vi "CreerReference.vi"() -> ()   [LabVIEW 2012]
panel:
  in  "Numéro":i32
  in  "stop":bool
  in  "Adresse du PilMOT":string="ni.var.psp://localhost/OPC/OPC1/esbimETH_1"
  in  "Move to ref":bool
  in  "Set":bool
  out "error out":errorcluster caption="sortie d'erreur"
  in  "error in (no error)":errorcluster caption="entrée d'erreur (pas d'erreur)"
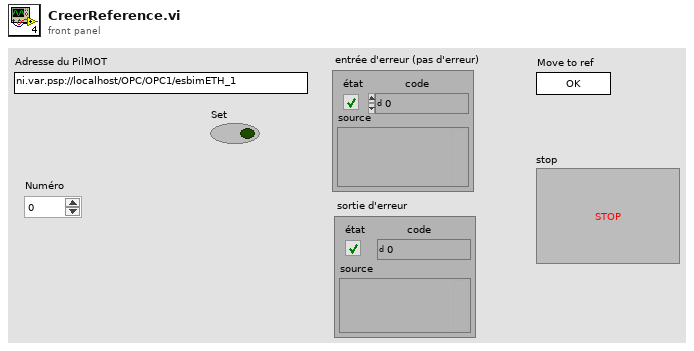
[diagram p1: front panel]
types:
  T1 = typedef "AdressesVariablesPartagees.ctl" = cluster{"OrdreBloc":string, "Ordre UC":string, "CoteAAtteindre":string, "Vitesse":string, "Position codeur en pas":string, "Position Théorique":string, "Message":string, "Ecrire":string, "Zone à écrire":string, "Numéro paramètre":string, "Ordre":string, "Valeur":string, "Valeur Lecture":string, "Numéro paramètre Lecture":string, "Acquittement Lecture Ecriture":string, "Zone à Ecrire Pour Axe ":u16, "Acquittement Ordre UC":string}
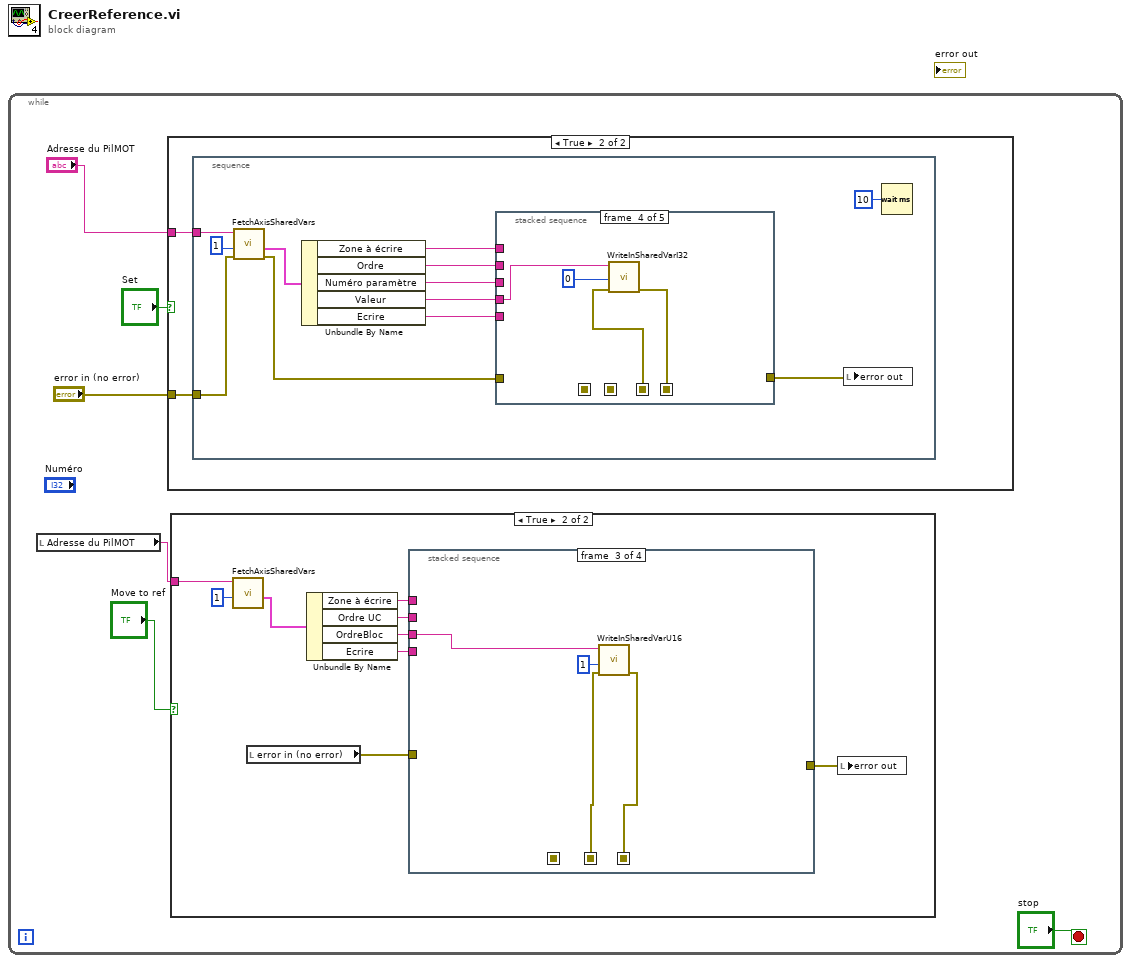
[diagram p0: block diagram]
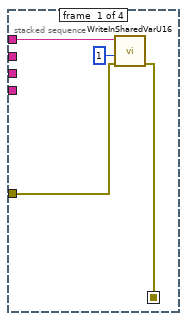
[diagram p3: hidden frame]
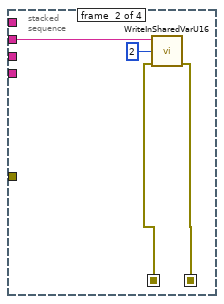
[diagram p4: hidden frame]
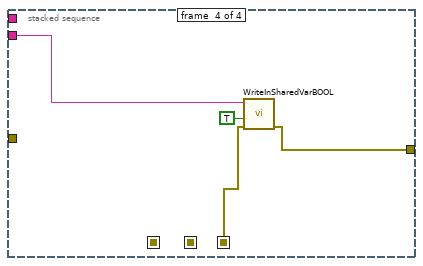
[diagram p5: hidden frame]
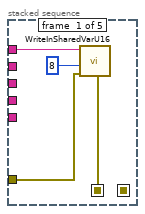
[diagram p7: hidden frame]
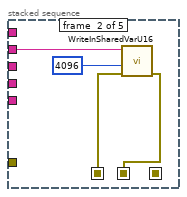
[diagram p8: hidden frame]
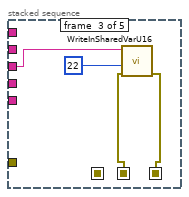
[diagram p9: hidden frame]
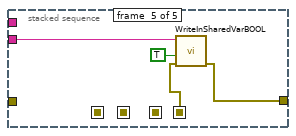
[diagram p10: hidden frame]
diagram:
  n1 = while {
    stop <- "stop" stop-if-true
    n2 = local read "Adresse du PilMOT"() -> (w2:string)
    n3 = case shown="True" "Set" {
      tunnel: "error in (no error)" -> [_ w33]
      tunnel: "Adresse du PilMOT" -> [_ w32]
      frame False {
      }
      frame True {
        n4 = stacked-sequence {
          tunnel: w33 -> [w45]
          tunnel: w32 -> [w44]
          frame #0 {
            n5 = call "FetchAxisSharedVars.vi"("error in (no error)"=w45, "Numéro d'Axe"=u32 1, "PilMOT Address"=w44) -> ("error out"=w36:errorcluster, "Sortie Variables d'Axes"=w37:T1)  [unwired: 7 in]
            n6 = Unbundle By Name(w37) -> ("Zone à écrire"=w43:string, "Ordre"=w42:string, "Numéro paramètre"=w41:string, "Valeur"=w40:string, "Ecrire"=w39:string)
            n7 = stacked-sequence {
              seq-local: [w47 _ _ _ _] -> [_ w52 _ _ _]
              seq-local: [_ w51 _ _ _] -> [_ _ w56 _ _]
              seq-local: [_ _ w54 _ _] -> [_ _ _ w61 _]
              seq-local: [_ _ _ w58 _] -> [_ _ _ _ w62]
              tunnel: w43 -> [w49 _ _ _ _]
              tunnel: w42 -> [_ w53 _ _ _]
              tunnel: w36 -> [w46 _ _ _ _]
              tunnel: w41 -> [_ _ w55 _ _]
              tunnel: w40 -> [_ _ _ w59 _]
              tunnel: w39 -> [_ _ _ _ w65]
              tunnel: [_ _ _ _ w63] -> w35
              frame #0 {
                n8 = call "WriteInSharedVarU16.vi"("entrée d'erreur (pas d'erreur)"=w46, "données en entrée"=u16 8, "refnum de variable partagée en entrée"=w49) -> ("sortie d'erreur"=w47:errorcluster)  [unwired: 8 in]
              }
              frame #1 {
                n9 = call "WriteInSharedVarU16.vi"("entrée d'erreur (pas d'erreur)"=w52, "données en entrée"=u16 4096, "refnum de variable partagée en entrée"=w53) -> ("sortie d'erreur"=w51:errorcluster)  [unwired: 8 in]
              }
              frame #2 {
                n10 = call "WriteInSharedVarU16.vi"("entrée d'erreur (pas d'erreur)"=w56, "données en entrée"=u16 22, "refnum de variable partagée en entrée"=w55) -> ("sortie d'erreur"=w54:errorcluster)  [unwired: 8 in]
              }
              frame #3 {
                n11 = call "WriteInSharedVarI32.vi"("entrée d'erreur (pas d'erreur)"=w61, "données en entrée"=0, "refnum de variable partagée en entrée"=w59) -> ("sortie d'erreur"=w58:errorcluster)  [unwired: 8 in]
              }
              frame #4 {
                n12 = call "WriteInSharedVarBOOL.vi"("entrée d'erreur (pas d'erreur)"=w62, "données en entrée"=TRUE, "refnum de variable partagée en entrée"=w65) -> ("sortie d'erreur"=w63:errorcluster)  [unwired: 8 in]
              }
            }
            n13 = local write "error out"(w35) -> ()
            n14 = Wait (ms)(milliseconds to wait=u32 10 ("attente (ms)")) -> ()  [unwired: 1 out]
          }
        }
      }
    }
    n15 = case shown="True" "Move to ref" {
      tunnel: w2 -> [_ w15]
      frame False {
      }
      frame True {
        n16 = call "FetchAxisSharedVars.vi"("Numéro d'Axe"=u32 1, "PilMOT Address"=w15) -> ("Sortie Variables d'Axes"=w13:T1)  [unwired: 8 in, 1 out]
        n17 = local read "error in (no error)"() -> (w11:errorcluster)
        n18 = Unbundle By Name(w13) -> ("Zone à écrire"=w12:string, "Ordre UC"=w10:string, "OrdreBloc"=w8:string, "Ecrire"=w9:string)
        n19 = stacked-sequence {
          seq-local: [w16 _ _ _] -> [_ w21 _ _]
          seq-local: [_ w20 _ _] -> [_ _ w25 _]
          seq-local: [_ _ w24 _] -> [_ _ _ w29]
          tunnel: w12 -> [w19 _ _ _]
          tunnel: w11 -> [w17 _ _ _]
          tunnel: w10 -> [_ w23 _ _]
          tunnel: w9 -> [_ _ _ w31]
          tunnel: w8 -> [_ _ w27 _]
          tunnel: [_ _ _ w28] -> w7
          frame #0 {
            n20 = call "WriteInSharedVarU16.vi"("entrée d'erreur (pas d'erreur)"=w17, "données en entrée"=u16 1, "refnum de variable partagée en entrée"=w19) -> ("sortie d'erreur"=w16:errorcluster)  [unwired: 8 in]
          }
          frame #1 {
            n21 = call "WriteInSharedVarU16.vi"("entrée d'erreur (pas d'erreur)"=w21, "données en entrée"=u16 2, "refnum de variable partagée en entrée"=w23) -> ("sortie d'erreur"=w20:errorcluster)  [unwired: 8 in]
          }
          frame #2 {
            n22 = call "WriteInSharedVarU16.vi"("entrée d'erreur (pas d'erreur)"=w25, "données en entrée"=u16 1, "refnum de variable partagée en entrée"=w27) -> ("sortie d'erreur"=w24:errorcluster)  [unwired: 8 in]
          }
          frame #3 {
            n23 = call "WriteInSharedVarBOOL.vi"("entrée d'erreur (pas d'erreur)"=w29, "données en entrée"=TRUE, "refnum de variable partagée en entrée"=w31) -> ("sortie d'erreur"=w28:errorcluster)  [unwired: 8 in]
          }
        }
        n24 = local write "error out"(w7) -> ()
      }
    }
  }
